vi "PicoScope5000aExampleBlockMSO.vi"() -> ()   [LabVIEW 2010]
uses:
  shared/PicoBuffers.ctl
  <vilib>/Waveform/DWDTOps.llb/DWDT Analog to Digital.vi
  PicoScope5000aLib/PicoScope5000aAnalogChannelSettings.ctl
  shared/Buffer and Transfer Settings.ctl
  shared/Acquisition Settings.ctl
  PicoScope5000aLib/PicoScope5000aDigitalChannelSettings.ctl
panel:
  out "overflow":i16 format="%010b"
  in  "Apply Settings":bool
  in  "Port 0 Settings":T1={"Enabled"=FALSE, "Logic Level"=9830} {"Logic Level" items=["1.5V TTL"=9830, "2.5V CMOS"=16383]}
  in  "Channel A Settings":T2={"Enabled"=TRUE, "Coupling"=1, "Range"=6, "Analogue Offset"=0.0, "Bandwidth Limit"=0} {"Bandwidth Limit" items=["Full", "20MHz"]; "Range" items=["10 mV", "20 mV", "50 mV", "100 mV", "200 mV", "500 mV", "1 V", "2 V", "5 V", "10 V", "20 V"]; "Coupling" items=["AC", "DC"]}
  in  "Trigger Settings":T3={"Trigger Enabled"=FALSE, "Trigger Source"=enum."Channel A", "Trigger Threshold (volts)"=0.0, "Trigger Direction"=2, "Trigger Delay (samples)"=0, "Auto Trigger Time (ms)"=1000} {"Trigger Direction" items=["Rising"=2, "Falling"=3]}
  out "USB 3.0 device on non-USB 3.0 Port":bool=TRUE
  out "USB Powered":bool=TRUE
  out "Device Info":T4={"Driver Version"="2.1.104.3324", "USB Version"="2.0", "Hardware"="1", "Variant"="5244A", "Batch and Serial"="CQ178/007", "Cal Date"="11Jun13", "Kernel Version"="1.0", "Digital HW Version"="1", "Analogue HW Version"="1", "MSO"=FALSE, "Number of channels"=2}
  out "error out":errorcluster
  in  "Data file":path=path "PicoScope5000aExampleBlock ChA Data"
  in  "Buffer and Transfer Settings":T5={"startIndex"=0, "Samples"=5000000, "Down Sample Ratio"=1, "Down-Sample Mode"=0} {"Down-Sample Mode" items=["RAW none"=2147483648, "None"=0, "Aggregate"=1, "Decimate"=2, "Average"=4]; "Down Sample Ratio" step=1; "Samples" format="%_6p"}
  in  "Acquisition Settings":T6={"preTriggerSamples"=0, "postTriggerSamples"=5000000, "timebase"=5} {"postTriggerSamples" format="%_6p"; "preTriggerSamples" format="%_6p"}
  out "Properties Panel":T7={"Sample Frequency"=41666668.0, "Sample Rate"=2.4000000209412065e-08, "Max Samples Available"=26843008, "Number of Samples"=0, "Total Capture Time (sec) "=0.0, "Max Total Capture Time Available (sec)"=0.6442322134971619} {"Max Total Capture Time Available (sec)" format="%.3p"; "Sample Frequency" format="%.6p"; "Sample Rate" format="%.3p"; "Max Samples Available" format="%_6p"; "Total Capture Time (sec)" format="%.3p"}
  out "Port 0":digitalwaveform(graph)={"t0"=timestamp(0 s since 1904-01-01), "dt"=8e-09, "Y"={"transitions"=[], "data"=[]}}
  in  "stop":bool
  out "Analog Channels":cluster{i32, sgl, "Data":dbl[]}[](graph)
  in  "Resolution":u32(ring) items=["8-bit"=0, "12-bit"=1, "14-bit"=2, "15-bit"=3, "16-bit"=4, "10-bit"=10]
  in  "Serial Number":string
  in  "Use Serial Number":bool
  in  "error in (no error)":errorcluster
  # "Bit 0 = ChA"
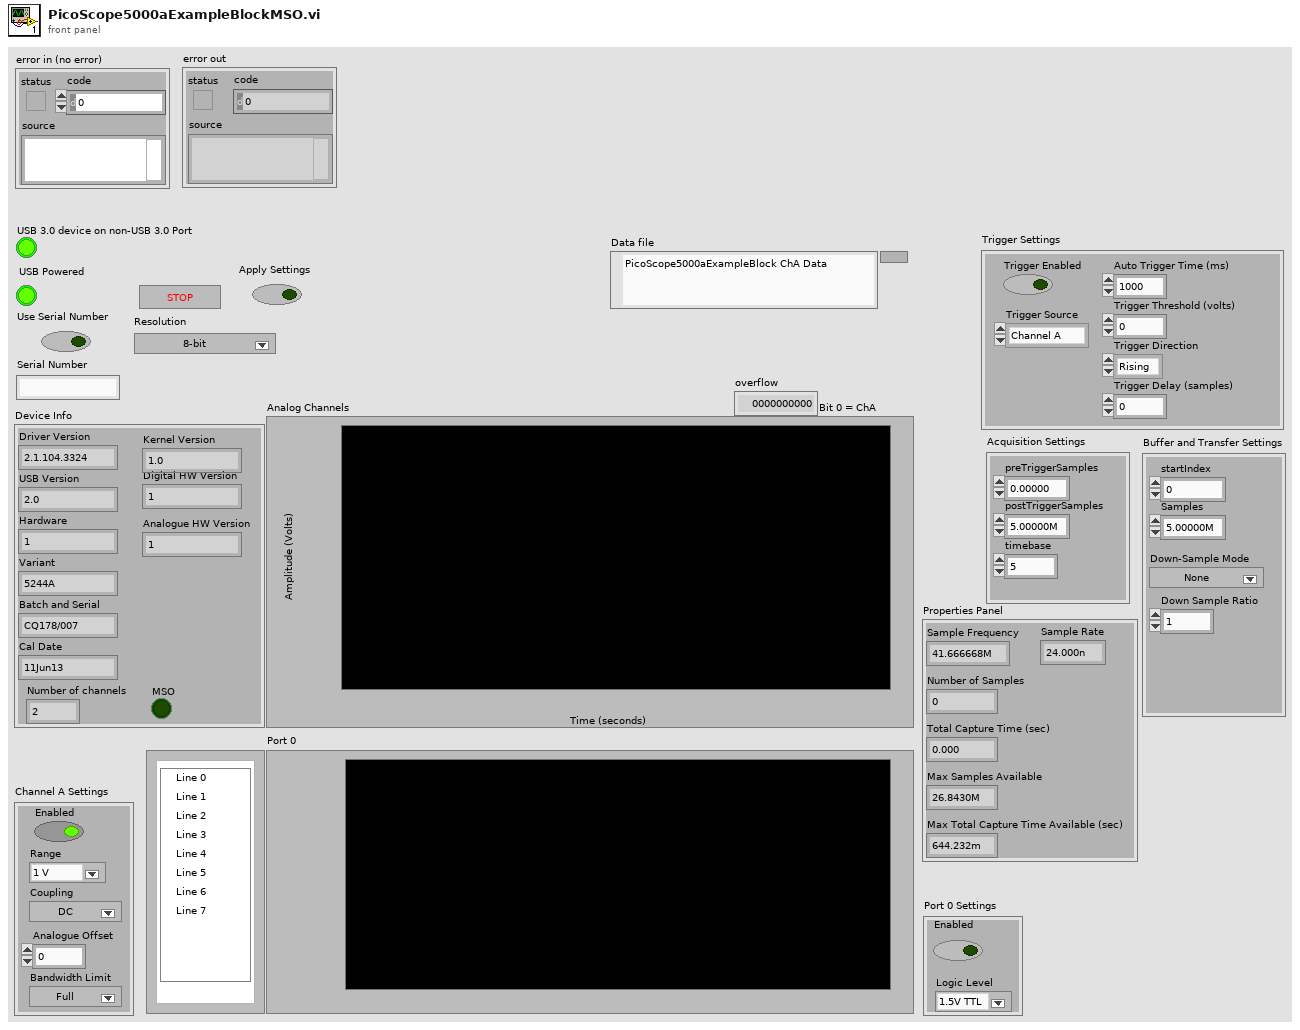
[diagram p1: front panel]
types:
  T1 = typedef "PicoScope5000aDigitalChannelSettings.ctl" = cluster{"Enabled":bool, "Logic Level":i16}
  T2 = typedef "PicoScope5000aAnalogChannelSettings.ctl" = cluster{"Enabled":bool, "Coupling":i16, "Range":u16, "Analogue Offset":sgl, "Bandwidth Limit":u32}
  T3 = cluster{"Trigger Enabled":bool, "Trigger Source":enum16{"Channel A", "Channel B", "Channel C", "Channel D", "Ext."}, "Trigger Threshold (volts)":dbl, "Trigger Direction":u16, "Trigger Delay (samples)":u32, "Auto Trigger Time (ms)":i16}
  T4 = cluster{"Driver Version":string, "USB Version":string, "Hardware":string, "Variant":string, "Batch and Serial":string, "Cal Date":string, "Kernel Version":string, "Digital HW Version":string, "Analogue HW Version":string, "MSO":bool, "Number of channels":i16}
  T5 = typedef "Buffer and Transfer Settings.ctl" = cluster{"startIndex":u64, "Samples":u64, "Down Sample Ratio":u64, "Down-Sample Mode":u32}
  T6 = typedef "Acquisition Settings.ctl" = cluster{"preTriggerSamples":u64, "postTriggerSamples":u64, "timebase":u32}
  T7 = cluster{"Sample Frequency":dbl, "Sample Rate":dbl, "Max Samples Available":u64, "Number of Samples":u64, "Total Capture Time (sec) ":dbl, "Max Total Capture Time Available (sec)":dbl}
  T8 = enum16{"open", "open or create", "create or replace", "create", "open (read-only)"}
  T9 = typedef "PicoBuffers.ctl" = cluster{"Max Buffer Pointers":u64[][][], "Min Buffer Pointers":u64[][][], "StreamingDataInfo":cluster{"Channel":u32, "Down-Sample Mode":u32, "PICO_DATA_TYPE":enum32{"PICO_INT8_T", "PICO_INT16_T", "PICO_INT32_T", "PICO_UINT32_T", "PICO_INT64_T", ""}, "Samples":i32, "bufferIndex":u64, "startIndex":i32, "overflow":i16}[][]}
  T10 = cluster{"Sample Frequency":sgl, "Sample Rate":sgl, "Max Samples Available":i32, "Number of Samples":u32, "Total Capture Time (sec) ":sgl, "Max Total Capture Time Available (sec)":sgl}
  T11 = cluster{"Channel A Buffer":i16[], "Channel B Buffer":i16[], "Channel C Buffer":i16[], "Channel D Buffer":i16[], "Channel E Buffer":i16[], "Channel F Buffer":i16[], "Channel G Buffer":i16[], "Channel H Buffer":i16[], "Port 0 Buffer":i16[], "Port 1 Buffer":i16[]}[]
  T12 = cluster{"Channel A Buffer":i16[], "Channel B Buffer":i16[], "Channel C Buffer":i16[], "Channel D Buffer":i16[], "Channel E Buffer":i16[], "Channel F Buffer":i16[], "Channel G Buffer":i16[], "Channel H Buffer":i16[], "Port 0 Buffer":i16[], "Port 1 Buffer":i16[]}
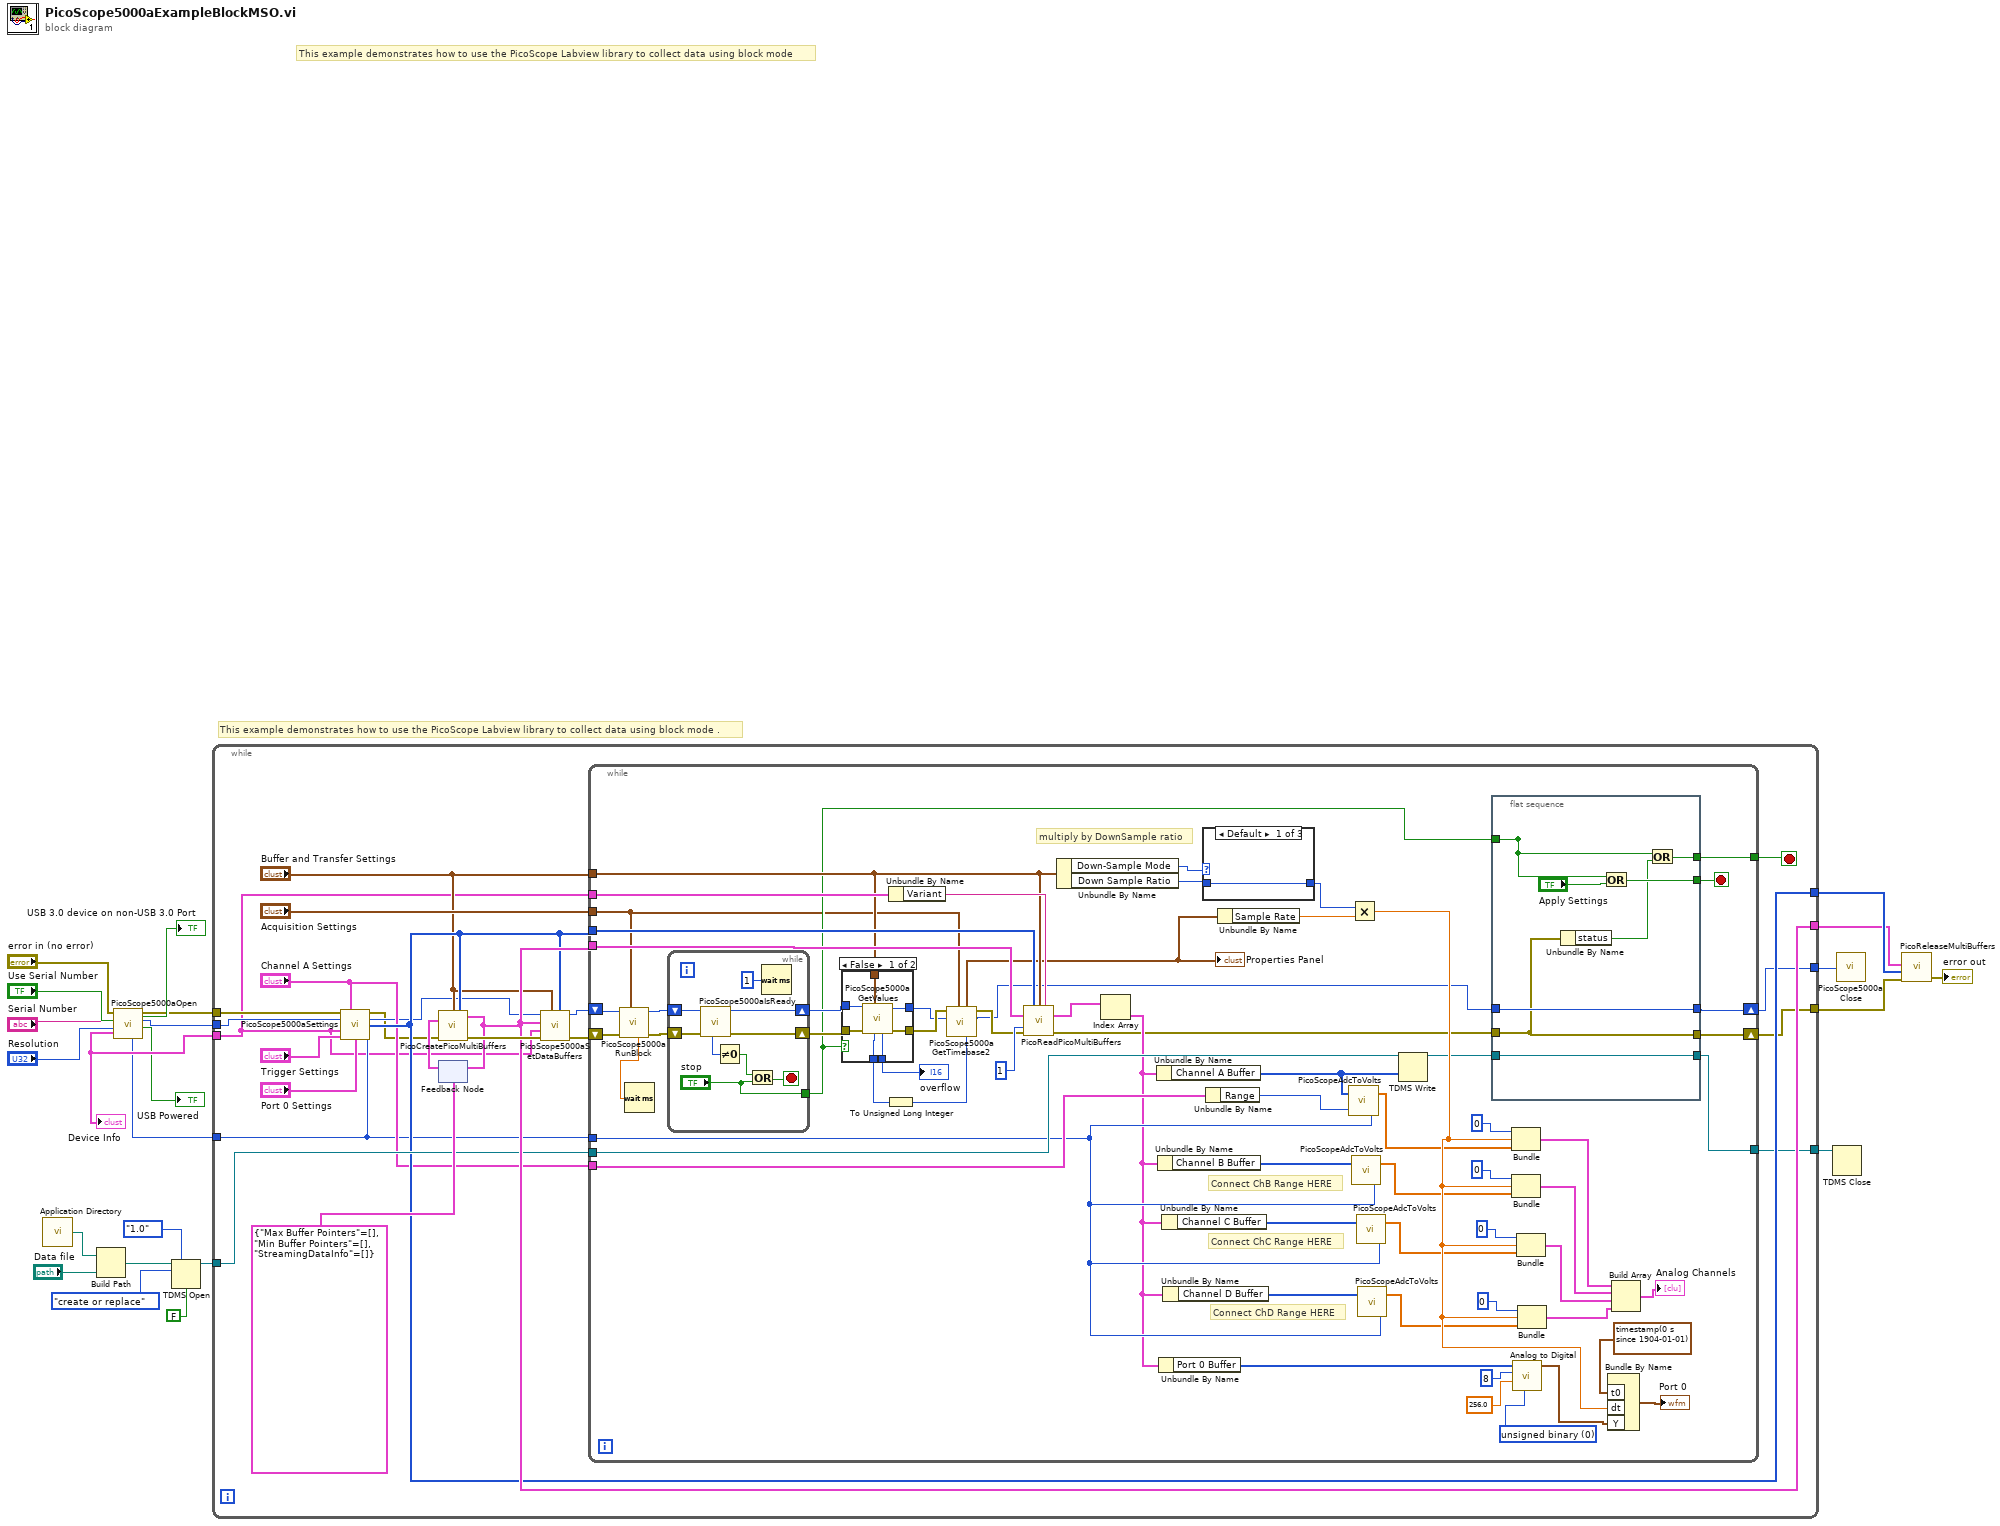
[diagram p0: block diagram]
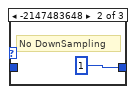
[diagram p3: hidden frame]
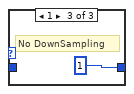
[diagram p4: hidden frame]
diagram:
  # "This example demonstrates how to use the PicoScope Labview library to collect data using block mode ."
  # "This example demonstrates how to use the PicoScope Labview library to collect data using block mode"
  n1 = call <vilib>:"Application Directory.vi"() -> ("Application Directory"=w15:path)
  n2 = Build Path(base path=w15, name or relative path="Data file") -> (appended path=w16:path)
  n3 = call "PicoScope5000aOpen.vi"("Serial Number"="Serial Number", "Resolution"="Resolution", "Use Serial Number"="Use Serial Number", "error in (no error)"="error in (no error)") -> ("USB Powered"=→"USB Powered":bool, "handle"=w23:i16, "error out"=w3:errorcluster, "Max ADC value"=w6:i16, "USB 3.0 device on non-USB 3.0 Port"=→"USB 3.0 device on non-USB 3.0 Port":bool, "Device Info"=w7:T4)  [unwired: 2 in]
  "Device Info" <- w7
  n4 = TDMS Open(6:FALSE ("disable buffering? (T)"), 7:enum16{"1.0", "2.0"}."1.0" ("file format version (2.0)"), 10:T8."create or replace" ("operation (0:open)"), 11:w16) -> (3:w13:refnum<k34>)  [unwired: 2 in, 1 out]
  n5 = while {
    tunnel: w23 -> [w41]
    tunnel: w6 -> [w34]
    tunnel: [w38] -> w22
    tunnel: [w43] -> w21
    tunnel: [w32] -> w14
    tunnel: w13 -> [w42]
    tunnel: w7 -> [w24]
    tunnel: w3 -> [w40]
    tunnel: [w33] -> w2
    tunnel: [w30] -> w1
    stop <- w31 stop-if-true
    n6 = call "PicoScope5000aSettings.vi"("error in"=w40, "Channel A Settings"="Channel A Settings", "Port 0 Settings"="Port 0 Settings", "handle in"=w41, "Device Info"=w24, "Trigger Settings"="Trigger Settings", "Max ADC value"=w34) -> ("error out"=w25:errorcluster, "handle out"=w26:i16, "enabled array"=w38:i16[])  [unwired: 6 in]
    n7 = feedback #1(T9 {"Max Buffer Pointers"=[], "Min Buffer Pointers"=[], "StreamingDataInfo"=[]} ("Data Pointers")) -> (w45:T9)
    n8 = call "PicoCreatePicoMultiBuffers.vi"("Buffer and Transfer Settings"="Buffer and Transfer Settings", "enabled array"=w38, "Data Pointers In"=w45, "error in (no error)"=w25) -> ("Data Pointers"=w43:T9, "error out"=w44:errorcluster)  [unwired: 10 in]
    n9 = feedback-in #1(w43) -> ()
    n10 = call "PicoScope5000aSetDataBuffers.vi"("enabled array"=w38, "Buffer and Transfer Settings"="Buffer and Transfer Settings", "error in (no error)"=w44, "Device Info"=w24, "Data Pointers In"=w43, "handle in"=w26) -> ("error out"=w29:errorcluster, "handle out"=w28:i16)  [unwired: 4 in]
    n11 = while {
      tunnel: w43 -> [w111]
      tunnel: "Buffer and Transfer Settings" -> [w58]
      tunnel: w38 -> [w102]
      tunnel: "Channel A Settings" -> [w101]
      tunnel: "Acquisition Settings" -> [w50]
      tunnel: w34 -> [w100]
      tunnel: w24 -> [w97]
      tunnel: [w65] -> w31
      shift-right: [w69] -> w33
      shift-left: w29 -> [w59]
      shift-right: [w63] -> w30
      shift-left: w28 -> [w60]
      tunnel: w42 -> [w110]
      tunnel: [w67] -> w32
      stop <- w64 stop-if-true
      w86 = u16 0 items=["unsigned binary", "offset binary", "2's complement"] ("data format (offset binary)")
      # "Connect ChB Range HERE"
      # "Connect ChD Range HERE"
      # "Connect ChC Range HERE"
      # "multiply by DownSample ratio"
      n12 = call "PicoScope5000aRunBlock.vi"("Acquisition Settings"=w50, "error in (no error)"=w59, "handle in"=w60) -> ("error out"=w104:errorcluster, "handle out"=w103:i16, "timeIndisposedMs"=w49:dbl)  [unwired: 5 in, 1 out]
      n13 = Wait (ms)(milliseconds to wait=w49) -> ()  [unwired: 1 out]
      n14 = while {
        shift-right: [w136] -> w61
        shift-left: w104 -> [w137]
        shift-right: [w135] -> w62
        shift-left: w103 -> [w134]
        tunnel: ["stop"] -> w57
        stop <- w131 stop-if-true
        n15 = call "PicoScope5000aIsReady.vi"("error in (no error)"=w137, "handle in"=w134) -> ("error out"=w136:errorcluster, "handle out"=w135:i16, "ready"=w133:i16)  [unwired: 7 in]
        n16 = Not Equal To 0?(x=w133) -> (x != 0?=w132:bool)
        n17 = Or(x=w132, y="stop") -> (x .or. y?=w131:bool)
        n18 = Wait (ms)(milliseconds to wait=u32 1) -> ()  [unwired: 1 out]
      }
      n19 = case shown="False" w57 {
        tunnel: w61 -> [w118 w119]
        tunnel: w62 -> [w117 w120]
        tunnel: [w116 w120] -> w54
        tunnel: [w115 w119] -> w55
        tunnel: w58 -> [w114 _]
        tunnel: [w113 _] -> w56
        tunnel: [w112 _] -> w48
        frame False {
          n20 = call "PicoScope5000aGetValues.vi"("Buffer and Transfer Settings"=w114, "error in (no error)"=w118, "handle in"=w117) -> ("error out"=w115:errorcluster, "handle out"=w116:i16, "overflow"=w113:i16, "noOfSamples"=w112:u64)  [unwired: 5 in]
        }
        frame True {
        }
      }
      "overflow" <- w56
      n21 = To Unsigned Long Integer(number=w48) -> (unsigned 32bit integer=w47:u32)
      n22 = Unbundle By Name(w97) -> ("Variant"=w98:string)
      n23 = call "PicoScope5000aGetTimebase2.vi"("Number of Samples"=w47, "Acquisition Settings"=w50, "handle in"=w54, "error in (no error)"=w55) -> ("handle out"=w52:i16, "error out"=w53:errorcluster, "Properties Panel"=w51:T10)  [unwired: 5 in]
      "Properties Panel" <- w51
      n24 = call "PicoReadPicoMultiBuffers.vi"("enabled array"=w102, "Buffer and Transfer Settings"=w58, "Variant"=w98, "Data Pointers"=w111, "No of Buffers"=1, "error in (no error)"=w53) -> ("MultiBuffers (Max or non-aggregated)"=w109:T11, "error out"=w66:errorcluster)  [unwired: 7 in, 1 out]
      n25 = Unbundle By Name(w58) -> ("Down-Sample Mode"=w107:u32, "Down Sample Ratio"=w108:u64)
      n26 = Index Array(array=w109) -> (element=w70:T12)  [unwired: 1 in]
      n27 = Unbundle By Name(w70) -> ("Channel A Buffer"=w79:i16[])
      n28 = Unbundle By Name(w70) -> ("Channel B Buffer"=w92:i16[])
      n29 = Unbundle By Name(w70) -> ("Port 0 Buffer"=w84:i16[])
      n30 = Unbundle By Name(w70) -> ("Channel C Buffer"=w77:i16[])
      n31 = Unbundle By Name(w70) -> ("Channel D Buffer"=w73:i16[])
      n32 = case shown="Default" w107 {
        tunnel: [w138 u64 1 ("Down Sample Ratio") u64 1 ("Down Sample Ratio")] -> w105
        tunnel: w108 -> [w138 _ _]
        frame Default {
        }
        frame -2147483648 {
          # "No DownSampling"
        }
        frame 1 {
          # "No DownSampling"
        }
      }
      n33 = Unbundle By Name(w101) -> ("Range"=w94:u16)
      n34 = Unbundle By Name(w51) -> ("Sample Rate"=w99:sgl)
      n35 = call "PicoScopeAdcToVolts.vi"("Max_adc"=w100, "Range Index"=w94, "Data"=w79) -> ("Data"=w80:dbl[])
      n36 = Multiply(x=w105, y=w99) -> (x*y=w106:sgl)
      n37 = call "PicoScopeAdcToVolts.vi"("Max_adc"=w100, "Data"=w92) -> ("Data"=w91:dbl[])  [unwired: 1 in]
      n38 = call "PicoScopeAdcToVolts.vi"("Max_adc"=w100, "Data"=w77) -> ("Data"=w76:dbl[])  [unwired: 1 in]
      n39 = call "PicoScopeAdcToVolts.vi"("Max_adc"=w100, "Data"=w73) -> ("Data"=w72:dbl[])  [unwired: 1 in]
      n40 = TDMS Write(0:w110, 9:w79) -> (4:w68:refnum<k34>)  [unwired: 4 in, 3 out]
      n41 = flat-sequence {
        tunnel: [w128] -> w64
        tunnel: [w121] -> _
        tunnel: [w125] -> w65
        tunnel: w52 -> [w124]
        tunnel: [w124] -> w63
        tunnel: w66 -> [w123]
        tunnel: [w123] -> w69
        tunnel: [w122] -> w67
        tunnel: w68 -> [w122]
        tunnel: w57 -> [w121]
        frame #0 {
          n42 = Unbundle By Name(w123) -> ("status"=w126:bool)
          n43 = Or(x=w121, y="Apply Settings") -> (x .or. y?=w128:bool)
          n44 = Or(x=w121, y=w126) -> (x .or. y?=w125:bool)
        }
      }
      n45 = Bundle(0, w106, "Data"=w80) -> (w90:cluster{i32, sgl, "Data":dbl[]})  [unwired: 1 in]
      n46 = Bundle(0, w106, "Data"=w91) -> (w89:cluster{i32, sgl, "Data":dbl[]})  [unwired: 1 in]
      n47 = call-poly <vilib>:"Analog to Digital.vi"("data format (offset binary)"=w86, "full-scale range (pk-pk)"=256.0, "resolution (16 bit)"=8, "analog waveform"=w84) -> ("digital waveform"=w81:digitalwaveform)  [unwired: 4 in, 3 out]
      n48 = Bundle(0, w106, "Data"=w76) -> (w75:cluster{i32, sgl, "Data":dbl[]})  [unwired: 1 in]
      n49 = Bundle(0, w106, "Data"=w72) -> (w71:cluster{i32, sgl, "Data":dbl[]})  [unwired: 1 in]
      n50 = Bundle By Name("t0"=timestamp(0 s since 1904-01-01), "dt"=w106, "Y"=w81) -> (→"Port 0":digitalwaveform)  [unwired: 1 in]
      n51 = Build Array(w90, w89, w75, w71) -> (→"Analog Channels":cluster{i32, sgl, "Data":dbl[]}[])
    }
  }
  n52 = TDMS Close(11:w14) -> ()  [unwired: 1 in, 2 out]
  n53 = call "PicoScope5000aClose.vi"("handle"=w1) -> ()
  n54 = call "PicoReleaseMultiBuffers.vi"("error in (no error)"=w2, "Enabled array"=w22, "Data Pointers"=w21) -> ("error out"=→"error out":errorcluster)  [unwired: 7 in, 1 out]
